vi "idn_action.vi"(0 "HGF_IMAQDevice":refnum<class "HGF_IMAQDevice.lvclass">, 5 "error in (no error)":errorcluster) -> (12 "resourceString":string, 13 "additionalInfo":string, 14 "HGF_IMAQDevice out":refnum<class "HGF_IMAQDevice.lvclass">, 15 "driverRevision":string="unknown", 16 "firmwareRevision":string="unknown", 17 "vendor":string="unknown", 18 "model":string="unknown", 19 "error out":errorcluster)   [LabVIEW 2014, in "HGF_IMAQ.lvlib" / "HGF_IMAQDevice.lvclass"]
doc: "This VI queries the current instrument firmware revision and instrument driver revision.\n\nFor detailed driver information including modification history, refer to the Readme file.\n\n<b>Hint:</b> This is a dynamic dispatch VI to be implemented by child classes."
uses:
  HGF_IMAQDevice.lvclass
  HGF_DeviceBaseClasses/HGF_DeviceBase/HGF_DeviceBase.lvclass
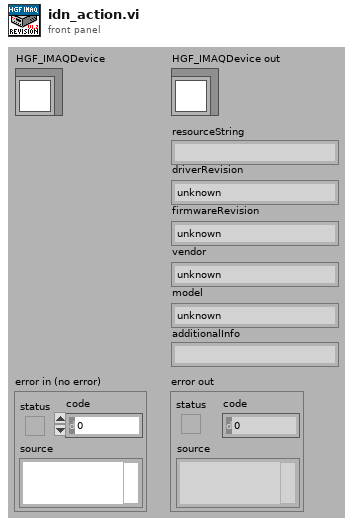
[diagram p1: front panel]
types:
  T1 = cluster{"Major":u16, "Minor":u16, "Fix":u16, "Build":u16}
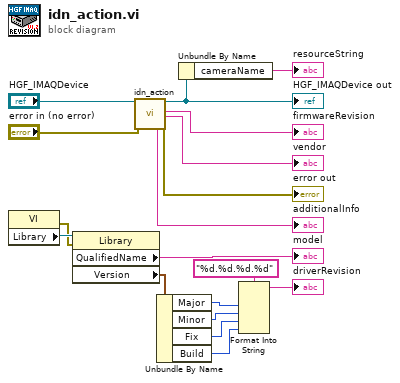
[diagram p0: block diagram]
diagram:
  n1 = property class="VI"() -> (error out=w3:errorcluster, "Library"=w4:refnum<vi>)  [unwired: 2 in, 1 out]
  n2 = property class="Library"(reference=w4, error in=w3) -> ("QualifiedName"=→"model":string, "Version"=w12:T1)  [unwired: 2 out]
  n3 = call-parent "idn_action.vi"("HGF_DeviceBase"="HGF_IMAQDevice", "error in (no error)"="error in (no error)") -> ("additionalInfo"=→"additionalInfo":string, "dup HGF_DeviceBase"=w2:refnum<class "HGF_IMAQDevice.lvclass">, "firmwareRevision"=→"firmwareRevision":string, "vendor"=→"vendor":string, "error out"=→"error out":errorcluster)  [unwired: 13 out]
  "HGF_IMAQDevice out" <- w2
  n4 = Unbundle By Name(w12) -> ("Major"=w11:u16, "Minor"=w10:u16, "Fix"=w9:u16, "Build"=w8:u16)
  n5 = Unbundle By Name(w2) -> ("cameraName"=→"resourceString":string)
  n6 = Format Into String(format string="%d.%d.%d.%d", w11, w10, w9, w8) -> (resulting string=→"driverRevision":string)  [unwired: 2 in, 1 out]
